vi "Angle2PMW.vi"(1 "Angle":dbl) -> (0 "PMW":u16)   [LabVIEW 2020]
panel:
  # "ГщнЯб уе уЮмб PMW"
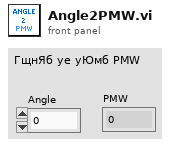
[diagram p1: front panel]
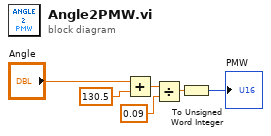
[diagram p0: block diagram]
diagram:
  n1 = Add(x="Angle", y=130.5) -> (x+y=w5:dbl)
  n2 = Divide(x=w5, y=0.09) -> (x/y=w1:dbl)
  n3 = To Unsigned Word Integer(number=w1) -> (unsigned 16bit integer=→"PMW":u16)
